vi "XYZ_set error.vi"   [LabVIEW 2023]
uses:
  <vilib>/NI/Modbus Library/API/Wrapper/Create Serial Master.vi
  <vilib>/NI/Modbus Library/API/master/Modbus Master.lvclass
  <vilib>/NI/Modbus Library/API/Wrapper/API Main.lvlib
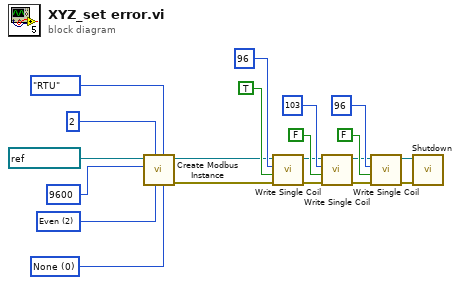
[diagram p0: block diagram]
diagram:
  w18 = u16 2 items=["None", "Odd", "Even", "Mark", "Space"] ("parity (even)")
  w20 = u16 0 items=["None", "XON/XOFF", "RTS/CTS", "XON/XOFF & RTS/CTS", "DTR/DSR", "XON/XOFF & DTR/DSR"] ("flow control (none)")
  n1 = call-poly <vilib>:"Create Modbus Instance.vi"("flow control (none)"=w20, "serial type"=enum16{"RTU", "ASCII"}."RTU", "parity (even)"=w18, "unit ID"=u8 2, "baud rate"=u32 9600, "VISA resource name"=refnum<visa-resource-name> "COM12") -> ("error out"=w7:errorcluster, "serial master instance"=w8:refnum<class "Modbus Master.lvclass">)  [unwired: 4 in]
  n2 = call-dynamic "Write Single Coil.vi"("error in"=w7, "coil to write"=TRUE, "address"=u16 96, "Modbus master in"=w8) -> ("error out"=w5:errorcluster, "Modbus master out"=w6:refnum<class "Modbus Master.lvclass">)  [unwired: 6 in]
  n3 = call-dynamic "Write Single Coil.vi"("error in"=w5, "coil to write"=FALSE, "address"=u16 103, "Modbus master in"=w6) -> ("error out"=w3:errorcluster, "Modbus master out"=w4:refnum<class "Modbus Master.lvclass">)  [unwired: 6 in]
  n4 = call-dynamic "Write Single Coil.vi"("error in"=w3, "coil to write"=FALSE, "address"=u16 96, "Modbus master in"=w4) -> ("error out"=w1:errorcluster, "Modbus master out"=w2:refnum<class "Modbus Master.lvclass">)  [unwired: 6 in]
  n5 = call-dynamic "Shutdown.vi"("error in"=w1, "Modbus master in"=w2) -> ()  [unwired: 9 in, 1 out]
